vi "detectAndSave.vi"() -> ()   [LabVIEW 2012]
uses:
  <vilib>/userdefined/High Color/IMAQdx.ctl
panel:
  out "image":T1(plugin-control)
  in  "image selector":u16(ring) items=["raw image", "single channel", "focus check", "downsampled", "subtraction result", "thresholded", "filtered", "cleaned", "cropped"]
  out "Number of Particles":i32
  out "Buffer Number Out":u32=569
  out "processed FPS":dbl=20.095693779904305
  out "acquired FPS":dbl=20.095693779904305
  in  "im proc controls":T2={"Color Plane"=2, "downsampling"=24, "Filter"=enum."AutoM", "Number of Erosions"=2, "Focus threshold"=20.0, "Focus std threshold"=0.0, "background\nsubtraction"=FALSE, "Threshold"=121} {"Threshold" scale=0.0..255.0; "Color Plane" items=["Red", "Green", "Blue", "Hue", "Saturation", "Luminance", "Value", "Intensity"]}
  in  "image format controls":T3={"Pixel Format"="YUV 422 Packed", "width"=2500, "height"=900, "sub image height"=2500, "sub image width"=2500}
  in  "camera controls":T5={"Camera Name"="cam0", "exposure time (us)"=10000, "GainRaw"=100, "Red balance"=64, "Green balance"=64, "Blue balance"=64}
  in  "stop":bool
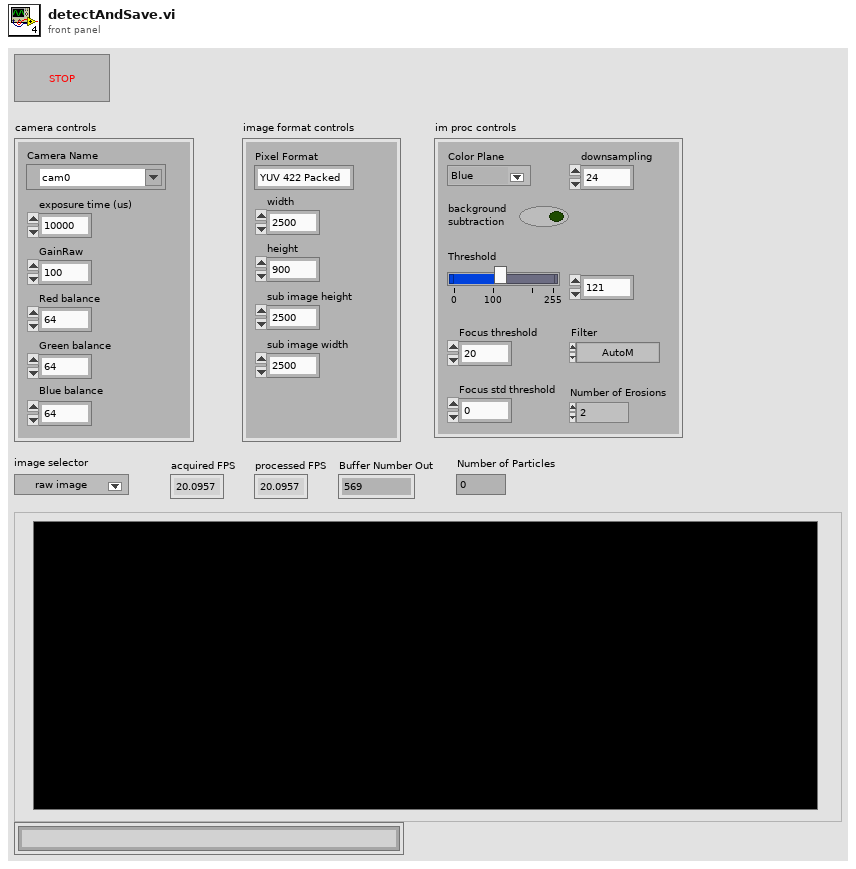
[diagram p1: front panel]
types:
  T1 = typedef "IMAQ Image.ctl" = refnum<image>
  T2 = cluster{"Color Plane":i32, "downsampling":i32, "Filter":enum32{"AutoM", "Close", "Dilate", "Erode", "Gradient", "Gradient out", "Gradient in", "Hit miss", "Open", "PClose", "POpen", "Thick", "Thin"}, "Number of Erosions":i32, "Focus threshold":sgl, "Focus std threshold":sgl, "background\nsubtraction":bool, "Threshold":u8}
  T3 = cluster{"Pixel Format":string, "width":u32, "height":u32, "sub image height":u32, "sub image width":u32}
  T4 = typedef "IMAQdx.ctl" = refnum<k21>
  T5 = cluster{"Camera Name":T4, "exposure time (us)":u32, "GainRaw":i64, "Red balance":u8, "Green balance":u8, "Blue balance":u8}
  T6 = cluster{"raw":T1, "single channel":T1, "focus check":T1, "downsampled":T1, "subtraction":T1, "thresholded":T1, "filtered":T1, "cleaned":T1, "cropped":T1}
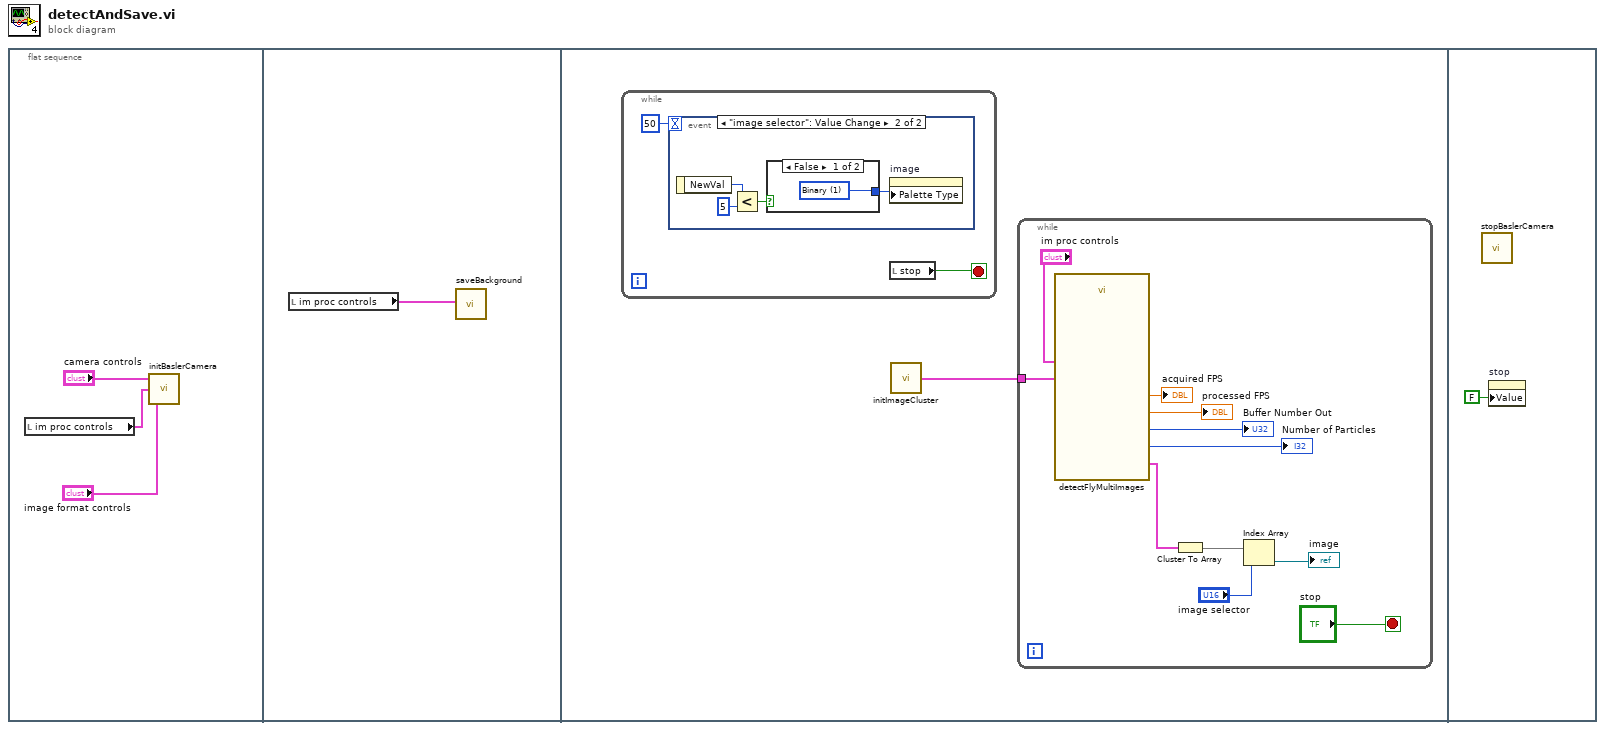
[diagram p0: block diagram]
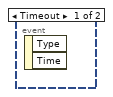
[diagram p2: hidden frame]
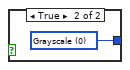
[diagram p3: hidden frame]
diagram:
  n1 = flat-sequence {
    frame #0 {
      n2 = local read "im proc controls"() -> (w1:T2)
      n3 = call "initBaslerCamera.vi"("camera controls"="camera controls", "im proc controls"=w1, "image format controls"="image format controls") -> ()  [unwired: 5 in]
    }
    frame #1 {
      n4 = local read "im proc controls"() -> (w4:T2)
      n5 = call "saveBackground.vi"("im proc controls"=w4) -> ()  [unwired: 11 in]
    }
    frame #2 {
      n6 = while {
        stop <- w6 stop-if-true
        n7 = event shown="[1] \"image selector\": Value Change" {
          selector: _ -> [_ _]
          dyn-events: _ -> [_ _]
          timeout: 50 -> [_ _]
          event Timeout {
            n8 = event-data() -> ()  [unwired: 1 in, 2 out]
          }
          event "image selector": Value Change {
            n9 = event-data() -> ("NewVal"=w11:u16)  [unwired: 1 in]
            n10 = Less?(x=w11, y=u16 5) -> (x < y?=w9:bool)
            n11 = case shown="False" w9 {
              tunnel: [w12 w13] -> w8
              frame False {
                w12 = u32 1 items=["Grayscale", "Binary", "Gradient", "Rainbow", "Temperature", "User Defined"] ("Palette:Palette Type")
              }
              frame True {
                w13 = u32 0 items=["Grayscale", "Binary", "Gradient", "Rainbow", "Temperature", "User Defined"] ("Palette:Palette Type")
              }
            }
            n12 = property on="image" class="ImageControl"("Palette Type"=w8) -> ()  [unwired: 2 in, 2 out]
          }
        }
        n13 = local read "stop"() -> (w6:bool)
      }
      n14 = call "initImageCluster.vi"() -> ("output cluster"=w5:T6)  [unwired: 5 in]
      n15 = while {
        tunnel: w5 -> [w22]
        stop <- "stop" stop-if-true
        n16 = call "detectFlyMultiImages.vi"("im proc controls"="im proc controls", "image cluster"=w22) -> ("acquired FPS"=→"acquired FPS":dbl, "processed FPS"=→"processed FPS":dbl, "Number of Particles"=→"Number of Particles":i32, "Buffer Number Out"=→"Buffer Number Out":u32, "image cluster out"=w17:T6)  [unwired: 9 in]
        n17 = Cluster To Array(cluster=w17) -> (array=w15:T1[])
        n18 = Index Array(array=w15, index="image selector") -> (element=→"image":T1)
      }
    }
    frame #3 {
      n19 = call "stopBaslerCamera.vi"() -> ()  [unwired: 12 in]
      n20 = property on="stop" class="Bool (strict)"("Value"=FALSE ("stop")) -> ()  [unwired: 2 in, 2 out]
    }
  }
